vi "NewCore.vi"(8 "error in (no error)":errorcluster, 10 "ParamsArray":variant[](array[variant]), 11 "MazeGame":refnum<class "EnchantedMazeGame.lvclass">) -> (0 "error out":errorcluster, 3 "MazeGame":refnum<class "EnchantedMazeGame.lvclass">)   [LabVIEW 2020, in "FactoryMethod.lvlib" / "NoParametrizedFactoryMethod.lvlib" / "EnchantedMazeGame.lvclass"]
uses:
  EnchantedMazeGame.lvclass
  Private/TypeDef/privateData.ctl
  EnchantedMazeGame.lvclass/EnchantedMazeGame.ctl
  MazeGame/MazeGame.lvclass
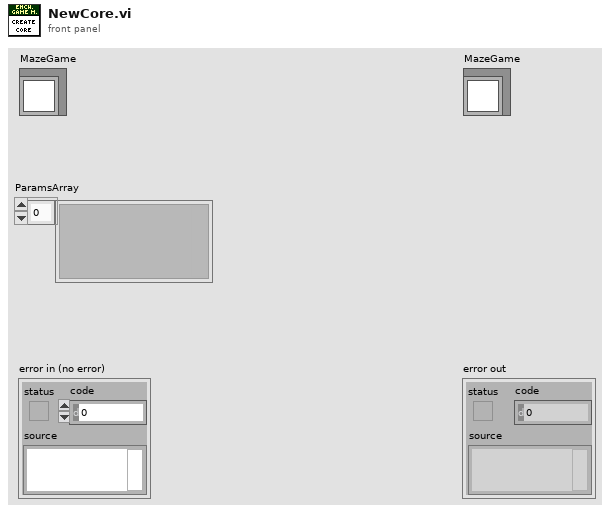
[diagram p1: front panel]
types:
  T1 = typedef "FactoryMethod.lvlib/NoParametrizedFactoryMethod.lvlib/EnchantedMazeGame.lvclass/privateData.ctl" = cluster{"Dummy":i32}
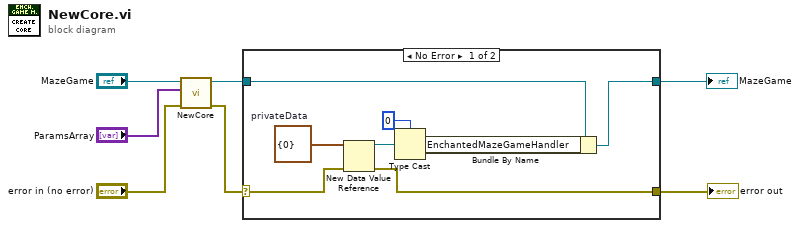
[diagram p0: block diagram]
diagram:
  n1 = call-parent "NewCore.vi"("error in (no error)"="error in (no error)", "ParamsArray"="ParamsArray", "MazeGame"="MazeGame") -> ("error out"=w1:errorcluster, "MazeGame"=w4:refnum<class "EnchantedMazeGame.lvclass">)  [unwired: 7 in]
  n2 = case shown="No Error" w1 {
    selector: w1 -> [w9 w17]
    tunnel: [w10 w17] -> w6
    tunnel: [w12 w16] -> w7
    tunnel: w4 -> [w11 w16]
    frame No Error {
      w8 = T1 {"Dummy"=0}  # privateData
      n3 = New Data Value Reference(data value=w8, error in=w9) -> (data value reference=w15:refnum<data-value>, error out=w10:errorcluster)
      n4 = Type Cast(type=u32 0, x=w15) -> (*(type *) &x=w13:u32)
      n5 = Bundle By Name(cluster=w11, "EnchantedMazeGameHandler"=w13) -> (w12:refnum<class "EnchantedMazeGame.lvclass">)
    }
    frame Error {
    }
  }
  "error out" <- w6
  "MazeGame" <- w7
